vi "HEWH ANSI Update Display.vi"(6 "Software Elapsed Time":dbl, 9 "ANSI Start Time":dbl, 10 "Absolute Pressure in":dbl, 11 "Stop Timer":dbl=1200.0 format="%#_13g") -> (1 "ANSI Display":string, 2 "Complete":bool, 3 "Absolute Pressure out":dbl, 4 "Raw Timer":dbl)   [LabVIEW 2023]
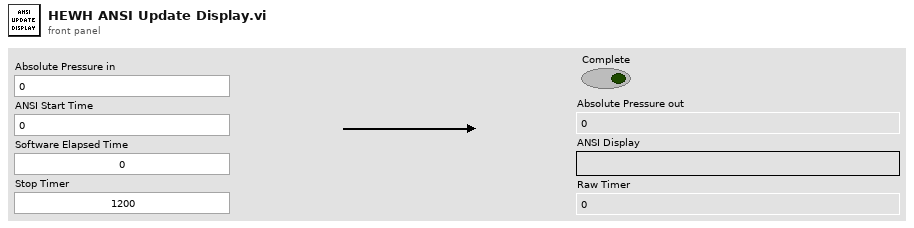
[diagram p1: front panel]
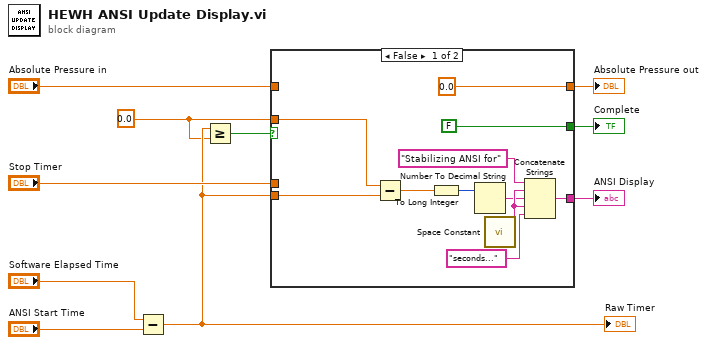
[diagram p0: block diagram]
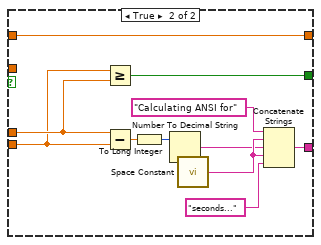
[diagram p2: hidden frame]
diagram:
  w1 = 0.0
  n1 = Subtract(x="Software Elapsed Time", y="ANSI Start Time") -> (x-y=w5:dbl)
  "Raw Timer" <- w5
  n2 = Greater Or Equal?(x=w5, y=w1) -> (x >= y?=w3:bool)
  n3 = case shown="False" w3 {
    tunnel: "Absolute Pressure in" -> [_ w32]
    tunnel: [0.0 ("ANSI Average (BTU/hr) Input") w32] -> w9
    tunnel: [w16 w25] -> w4
    tunnel: w1 -> [w14 _]
    tunnel: w5 -> [w13 w22]
    tunnel: [FALSE w24] -> w10
    tunnel: "Stop Timer" -> [_ w23]
    frame False {
      n4 = Subtract(x=w14, y=w13) -> (x-y=w12:dbl)
      n5 = To Long Integer(number=w12) -> (32bit integer=w15:i32)
      n6 = Number To Decimal String(number=w15) -> (decimal integer string=w18:string)  [unwired: 1 in]
      n7 = call <vilib>:"Space Constant.vi"() -> ("String"=w19:string)
      n8 = Concatenate Strings("Stabilizing ANSI for", w19, w18, w19, "seconds..." ("string")) -> (w16:string)
    }
    frame True {
      n9 = Greater Or Equal?(x=w22, y=w23) -> (x >= y?=w24:bool)
      n10 = Subtract(x=w23, y=w22) -> (x-y=w26:dbl)
      n11 = To Long Integer(number=w26) -> (32bit integer=w27:i32)
      n12 = Number To Decimal String(number=w27) -> (decimal integer string=w29:string)  [unwired: 1 in]
      n13 = call <vilib>:"Space Constant.vi"() -> ("String"=w30:string)
      n14 = Concatenate Strings("Calculating ANSI for", w30, w29, w30, "seconds..." ("string")) -> (w25:string)
    }
  }
  "ANSI Display" <- w4
  "Complete" <- w10
  "Absolute Pressure out" <- w9
